vi "BundleMagic TEST.vi"() -> ()   [LabVIEW 2023]
uses:
  <vilib>/Utility/miscctls.llb/LVBoundsTypeDef.ctl
  <vilib>/Utility/miscctls.llb/LVPositionTypeDef.ctl
panel:
  out "Position":T1
  in  "Ctl Refnum":refnum<vi>
  out "Cluster with unnamed elements 2":T2
  in  "Single Element Cluster":cluster{"Numeric":dbl}
  in  "Cluster with unnamed elements":T3
  in  "Cluster with Dotted Names":T4 {"C1.1"."N2.2" format="%.3p"}
  out "Bounds":T5
  out "Owner":refnum<vi>
  in  "Cluster":T6 {"C1"."N2" format="%.3p"}
  # "Dummy controls for use on BD"
  # "BundleMag!c FP Actions"
  # "Select Classes via Browse Classes... dialog on this control"
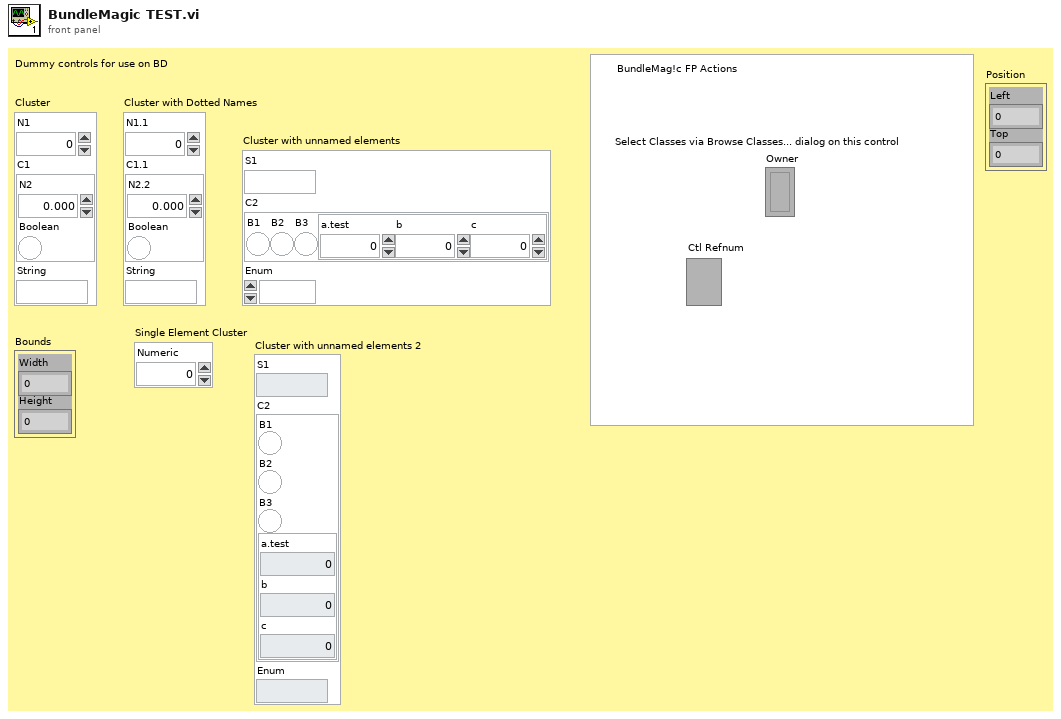
[diagram p1: front panel]
types:
  T1 = typedef "LVPositionTypeDef.ctl" = cluster{"Left":i32, "Top":i32}
  T2 = cluster{"S1":string, "C2":cluster{"B1":bool, "B2":bool, "B3":bool, "Cluster":cluster{"a.test":dbl, "b":i32, "c":u8}}, "Enum":enum16{""}}
  T3 = cluster{"S1":string, "C2":cluster{"B1":bool, "B2":bool, "B3":bool, cluster{"a.test":dbl, "b":i32, "c":u8}}, "Enum":enum16{""}}
  T4 = cluster{"N1.1":dbl, "C1.1":cluster{"N2.2":dbl, "Boolean":bool}, "String":string}
  T5 = typedef "LVBoundsTypeDef.ctl" = cluster{"Width":u32, "Height":u32}
  T6 = cluster{"N1":dbl, "C1":cluster{"N2":dbl, "Boolean":bool}, "String":string}
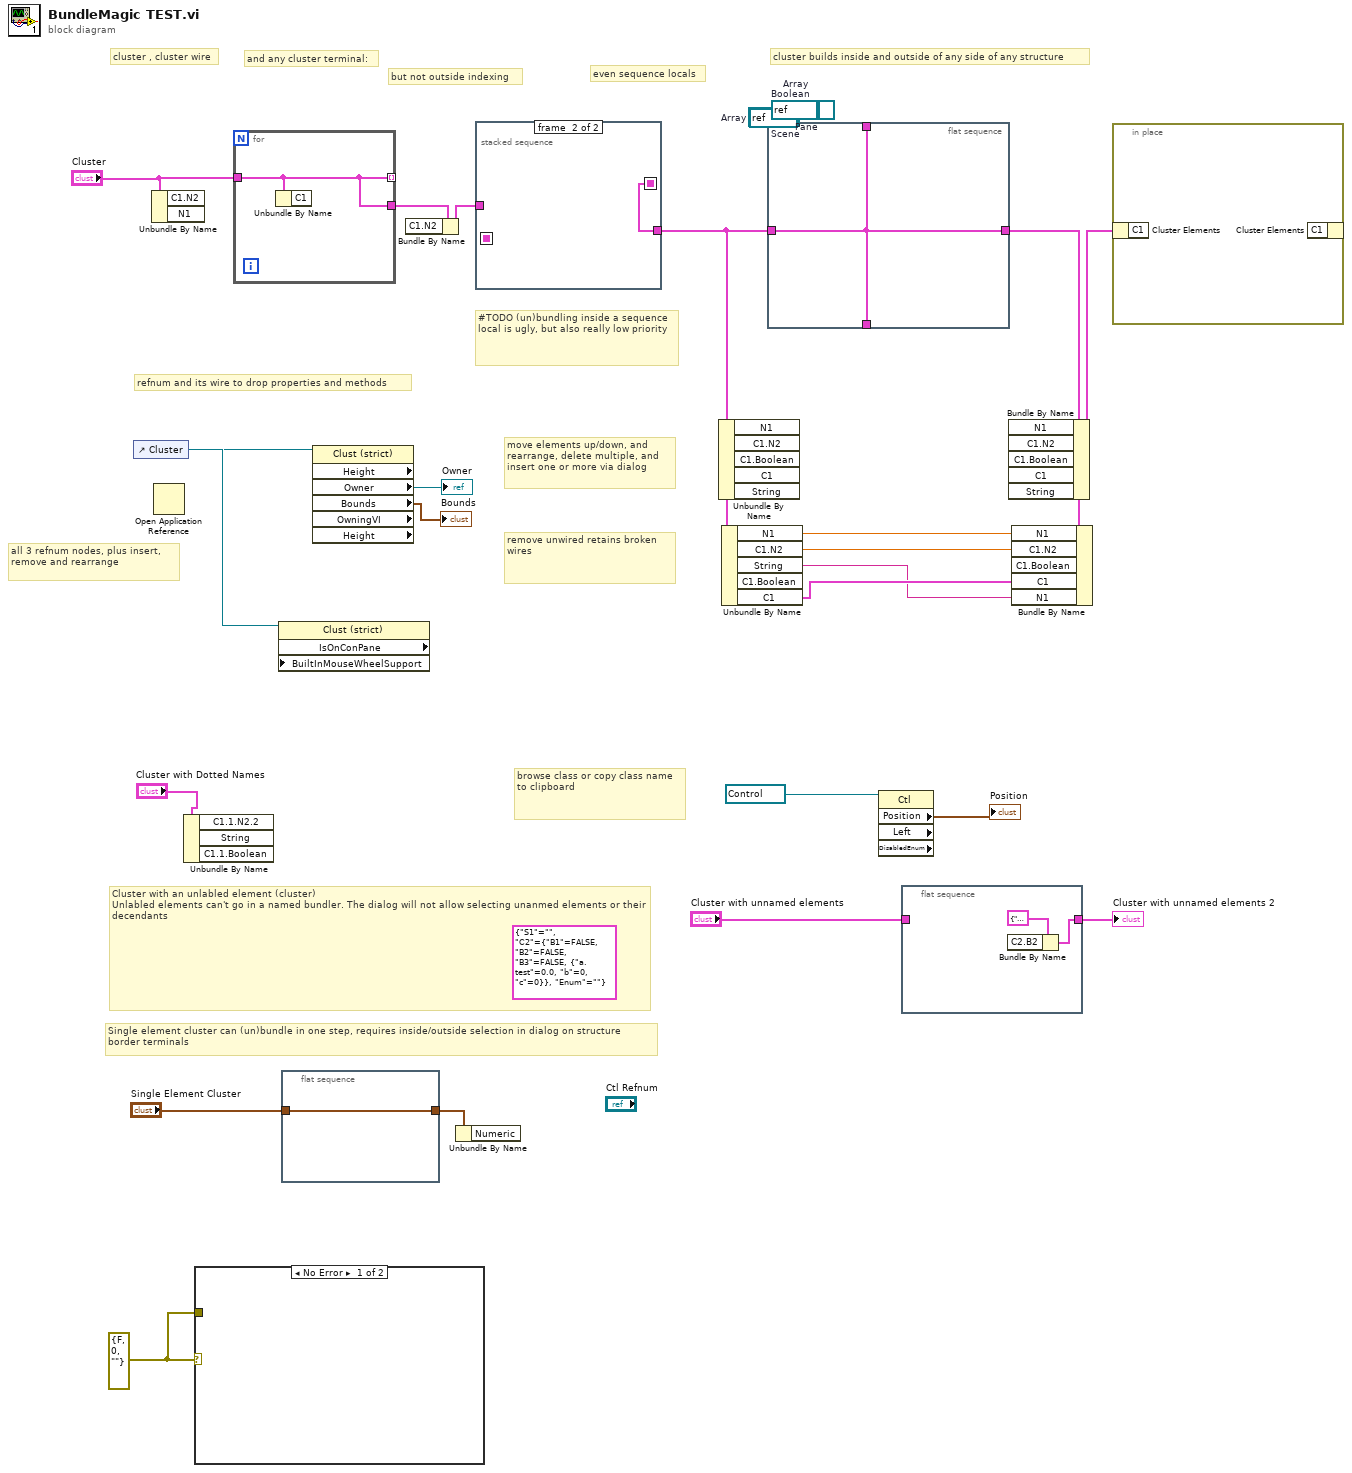
[diagram p0: block diagram]
diagram:
  (unwired) refnum<vi> refnum  # Boolean
  (unwired) refnum<vi> refnum  # Array
  (unwired) refnum<vi> refnum  # Pane
  (unwired) refnum<vi> refnum  # Scene
  (unwired) refnum<vi> refnum  # Array
  w4 = errorcluster {"status"=FALSE, "code"=0, "source"=""} ("error constant")
  (unwired) T3 {"S1"="", "C2"={"B1"=FALSE, "B2"=FALSE, "B3"=FALSE, {"a.test"=0.0, "b"=0, "c"=0}}, "Enum"=enum.""} ("C1")
  # "browse class or copy class name to clipboard"
  # "remove unwired retains broken wires"
  # "move elements up/down, and rearrange, delete multiple, and insert one or more via dialog"
  # "#TODO (un)bundling inside a sequence local is ugly, but also really low priority"
  # "even sequence locals"
  # "but not outside indexing"
  # "and any cluster terminal:"
  # "cluster , cluster wire"
  # "cluster builds inside and outside of any side of any structure"
  # "refnum and its wire to drop properties and methods"
  # "all 3 refnum nodes, plus insert, remove and rearrange"
  # "Cluster with an unlabled element (cluster)\nUnlabled elements can't go in a named bundler. The dialog will not allow selecting unanmed elements or their decendants"
  # "Single element cluster can (un)bundle in one step, requires inside/outside selection in dialog on structure border terminals"
  n1 = control-ref of="Cluster"() -> (w13:refnum<vi>)
  n2 = Unbundle By Name("Cluster") -> ()  [unwired: 2 out]
  n3 = Open Application Reference() -> ()  [unwired: 4 in, 2 out]
  n4 = Unbundle By Name("Cluster with Dotted Names") -> ()  [unwired: 3 out]
  n5 = case shown="No Error" w4 {
    tunnel: w4 -> [_ _]
    frame No Error {
    }
    frame Error {
    }
  }
  n6 = for {
    tunnel: [w28] -> _ mode=indexing
    tunnel: "Cluster" -> [w28]
    tunnel: [w28] -> w27
    n7 = Unbundle By Name(w28) -> ()  [unwired: 1 out]
  }
  n8 = property class="Clust (strict)" props=["IsOnConPane", "BuiltInMouseWheelSupport"](reference=w13) -> (reference out=w6:refnum<vi>)  [unwired: 2 in, 2 out]
  n9 = flat-sequence {
    tunnel: [w29] -> w2
    tunnel: "Single Element Cluster" -> [w29]
    frame #0 {
    }
  }
  n10 = property class="Clust (strict)" props=["Height", "Owner", "Bounds", "OwningVI", "Height"](reference=w6) -> ("Owner"=→"Owner":refnum<vi>, "Bounds"=→"Bounds":T5)  [unwired: 1 in, 5 out]
  n11 = Bundle By Name(cluster=w27) -> (w15:T6)  [unwired: 1 in]
  n12 = Unbundle By Name(w2) -> ()  [unwired: 1 out]
  n13 = stacked-sequence {
    seq-local: [w30 _] -> [_ w31]
    seq-local: [w30 _] -> [_ _]
    tunnel: w15 -> [w30 _]
    tunnel: [_ w31] -> w10
    frame #0 {
    }
    frame #1 {
    }
  }
  n14 = Unbundle By Name(w10) -> ()  [unwired: 5 out]
  n15 = Unbundle By Name(w10) -> ("N1"=w18:dbl, "C1.N2"=w19:dbl, "String"=w11:string, "C1"=w20:cluster{"N2":dbl, "Boolean":bool})  [unwired: 1 out]
  n16 = flat-sequence {
    tunnel: [w32] -> _
    tunnel: w10 -> [w32]
    tunnel: [w32] -> _
    tunnel: [w32] -> w9
    frame #0 {
    }
  }
  n17 = property class="Ctl" props=["Position", "Left", "DisabledEnum"](reference=refnum<vi> refnum ("Owner")) -> ("Position"=→"Position":T1)  [unwired: 1 in, 4 out]
  n18 = flat-sequence {
    tunnel: [w34] -> w12
    tunnel: "Cluster with unnamed elements" -> [_]
    frame #0 {
      n19 = Bundle By Name(cluster=T3 {"S1"="", "C2"={"B1"=FALSE, "B2"=FALSE, "B3"=FALSE, {"a.test"=0.0, "b"=0, "c"=0}}, "Enum"=enum.""} ("Cluster with unnamed elements")) -> (w34:T3)  [unwired: 1 in]
    }
  }
  n20 = Bundle By Name(cluster=w9) -> (w26:T6, "N1"=w25:dbl, "C1.N2"=w24:dbl, "C1.Boolean"=w22:bool, "C1"=w23:cluster{"N2":dbl, "Boolean":bool}, "String"=w21:string)
  n21 = Bundle By Name(cluster=w9, "N1"=w18, "C1.N2"=w19, "C1"=w20, "N1"=w11) -> ()  [unwired: 1 in, 1 out]
  n22 = in-place {
    n23 = in-place-cluster #1(w26) -> ()  [unwired: 1 out]
    n24 = in-place-cluster #1() -> ()  [unwired: 1 in, 1 out]
  }
  "Cluster with unnamed elements 2" <- w12
